vi "getTagRSSI.vi"(10 "Data Arry":u8[](array[numeric]) format="%x") -> (2 "RSSI":i32)   [LabVIEW 2018]
panel:
  # "Get Tag RSSI"
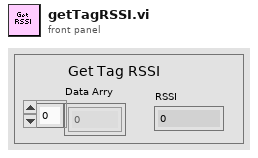
[diagram p1: front panel]
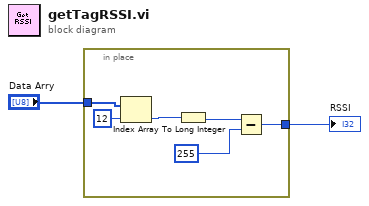
[diagram p0: block diagram]
diagram:
  n1 = in-place {
    in-place-border: "Data Arry" -> [w8]
    in-place-border: [w6] -> w1
    n2 = Index Array(array=w8, index=12) -> (element=w4:u8)
    n3 = To Long Integer(number=w4) -> (32bit integer=w3:i32)
    n4 = Subtract(x=w3, y=u8 255) -> (x-y=w6:i32)
  }
  "RSSI" <- w1
